vi "setRange.vi"(8 "Error In":errorcluster, 9 "maximum":i32, 10 "minimum":i32, 11 "QWinTaskbarProgress In":refnum<class "QWinTaskbarProgress.lvclass">) -> (0 "Error Out":errorcluster, 3 "QWinTaskbarProgress Out":refnum<class "QWinTaskbarProgress.lvclass">)   [LabVIEW 2014, in "QWinTaskbarProgress.lvclass"]
doc: "LabVIEW-specific documentation is not yet available. See <b>https://doc.qt.io/qt-5/qwintaskbarprogress.html#setRange</b>"
uses:
  QWinTaskbarProgress.lvclass
  LQ Core/LQIdentity/LQIdentity.lvclass/LQIdentity.ctl
  LQ Core/LQ Core.lvlib
  LQ Core/LQIdentity/LQIdentity.lvclass
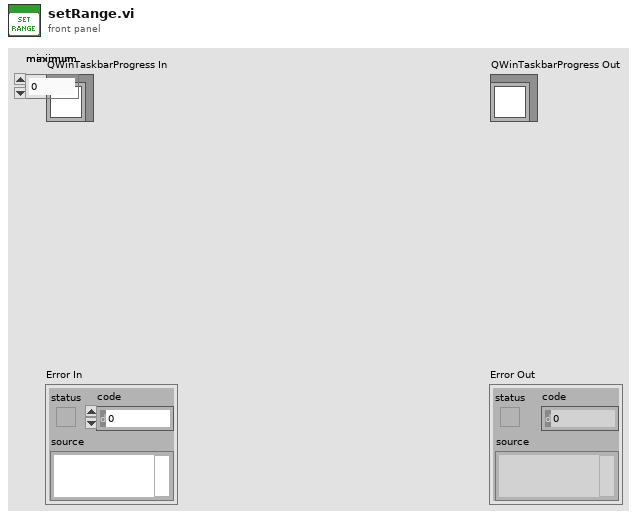
[diagram p1: front panel]
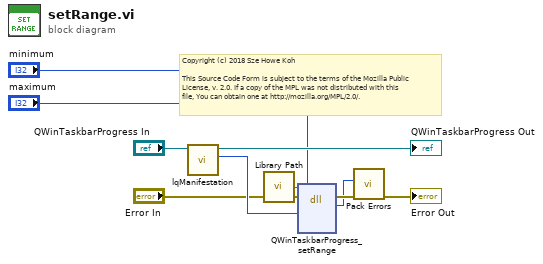
[diagram p0: block diagram]
diagram:
  # "Copyright (c) 2018 Sze Howe Koh\n\nThis Source Code Form is subject to the terms of the Mozilla Public\nLicense, v. 2.0. If a copy of the MPL was not distributed with this\nfile, You can obtain one at http://mozilla.org/MPL/2.0/."
  n1 = call "lqManifestation.vi"("LQIdentity in"="QWinTaskbarProgress In") -> ("Manifestation"=w7:u64, "LQIdentity out"=→"QWinTaskbarProgress Out":refnum<class "QWinTaskbarProgress.lvclass">)  [unwired: 9 in]
  n2 = call "Library Path.vi"() -> ("Library Path"=w8:path)
  n3 = dll-call lib="?" fn="QWinTaskbarProgress_setRange"(path in=w8, error in="Error In", "_instance"=w7, "minimum"="minimum", "maximum"="maximum") -> (error out=w5:errorcluster, w3:i32)  [unwired: 4 in, 1 out]
  n4 = call "Pack Errors.vi"("Error In"=w5, "Error Code"=w3) -> ("Error Out"=→"Error Out":errorcluster)  [unwired: 9 in]
